vi "TR_Set_List_Item_Value.vi"(8 "error in (no error)":errorcluster, 9 "Basic settings":variant, 10 "Track # in":i32, 11 "MulticolumnListbox in":refnum<vi>) -> (0 "error out":errorcluster, 3 "MulticolumnListbox out":refnum<vi>)   [LabVIEW 2018, in "Tracks Repair.lvlib"]
uses:
  Tracks Repair.lvlib
  SubVi's/Controls/CTL_Basic_cage_settings.ctl
  Tracker.lvlib
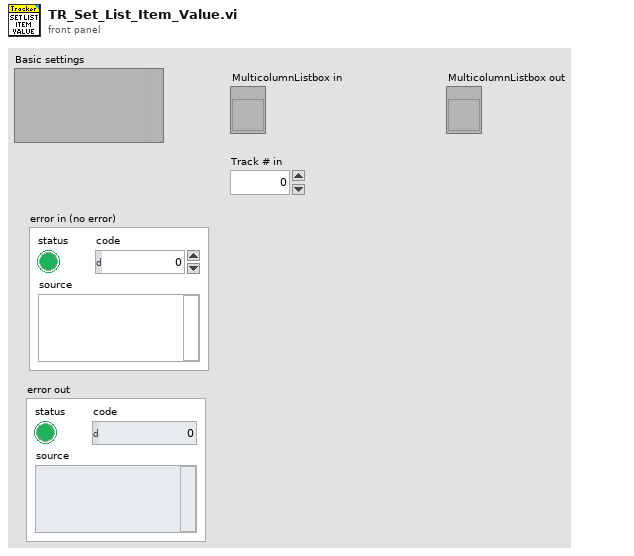
[diagram p1: front panel]
types:
  T1 = typedef "Tracker.lvlib/CTL_Basic_cage_settings.ctl" = cluster{"Vert. offset":dbl, "Hor. offset":dbl, "Bridge swap":bool, "Twisted neck":bool, "Cage diam.":i32, "Magn.rot.":i32, "Acq. speed":dbl}
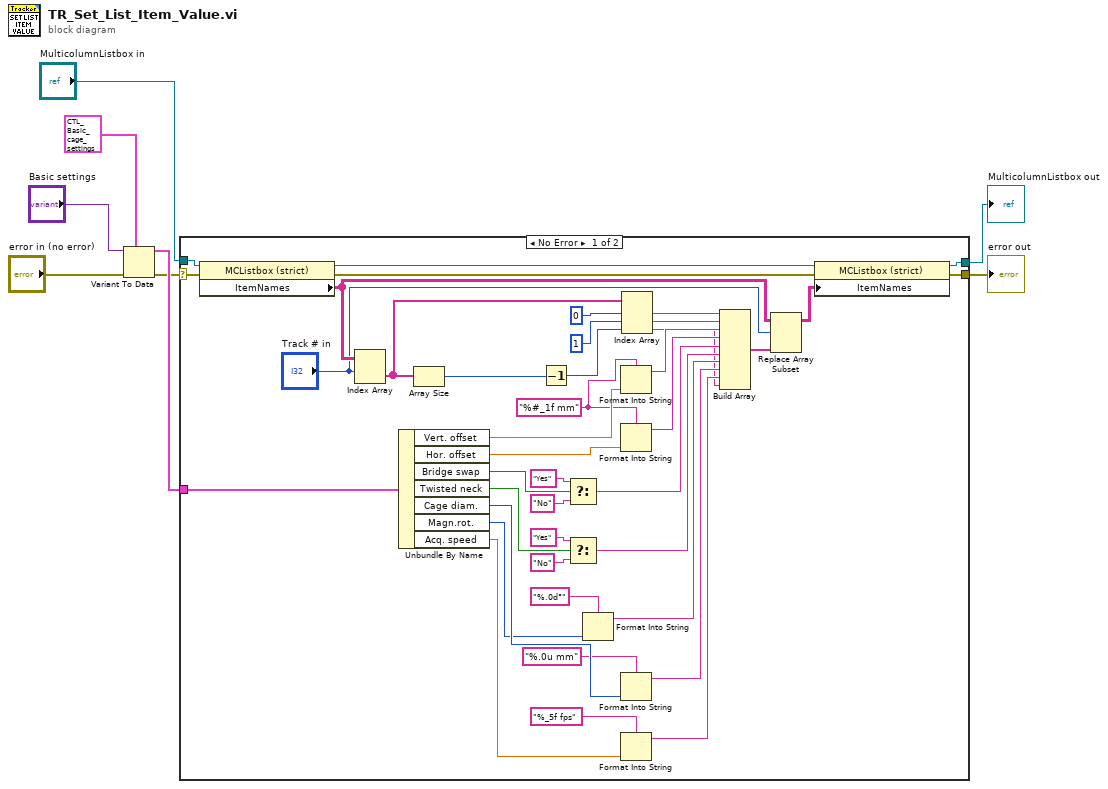
[diagram p0: block diagram]
diagram:
  n1 = Variant To Data(error in="error in (no error)", type=T1 {"Vert. offset"=10.0, "Hor. offset"=0.0, "Bridge swap"=FALSE, "Twisted neck"=FALSE, "Cage diam."=325, "Magn.rot."=0, "Acq. speed"=100.01280589338842} ("Basic settings"), Variant="Basic settings") -> (data=w6:T1, error out=w1:errorcluster)
  n2 = case shown="No Error" w1 {
    selector: w1 -> [w9 w51]
    tunnel: w6 -> [w27 _]
    tunnel: "MulticolumnListbox in" -> [w26 w50]
    tunnel: [w11 w51] -> w3
    tunnel: [w10 w50] -> w2
    frame No Error {
      w30 = "%#_1f mm" ("format string")
      n3 = property class="MCListbox (strict)"(reference=w26, error in=w9) -> (reference out=w13:refnum<vi>, error out=w14:errorcluster, "ItemNames"=w17:string[][])
      n4 = Index Array(array=w17, index (row)="Track # in") -> (element=w22:string[])  [unwired: 1 in]
      n5 = Unbundle By Name(w27) -> ("Vert. offset"=w49:dbl, "Hor. offset"=w47:dbl, "Bridge swap"=w45:bool, "Twisted neck"=w40:bool, "Cage diam."=w37:i32, "Magn.rot."=w35:i32, "Acq. speed"=w33:dbl)
      n6 = Array Size(array=w22) -> (size(s)=w25:i32)
      n7 = Decrement(x=w25) -> (x-1=w24:i32)
      n8 = Select(t="Yes", s=w45, f="No") -> (s? t:f=w39:string)
      n9 = Select(t="Yes", s=w40, f="No") -> (s? t:f=w38:string)
      n10 = Format Into String(format string="%.0d°", w35) -> (resulting string=w29:string)  [unwired: 2 in, 1 out]
      n11 = Format Into String(format string=w30, w49) -> (resulting string=w48:string)  [unwired: 2 in, 1 out]
      n12 = Format Into String(format string=w30, w47) -> (resulting string=w46:string)  [unwired: 2 in, 1 out]
      n13 = Format Into String(format string="%.0u mm", w37) -> (resulting string=w28:string)  [unwired: 2 in, 1 out]
      n14 = Format Into String(format string="%_5f fps", w33) -> (resulting string=w31:string)  [unwired: 2 in, 1 out]
      n15 = Index Array(array=w22, index #1=0 ("index (row)"), index #2=1 ("index"), index #3=w24) -> (element #1=w20:string, element #2=w19:string, element #3=w18:string)
      n16 = Build Array(w20, w19, w48, w46, w39, w38, w29, w28, w31, w18) -> (w15:string[])
      n17 = Replace Array Subset(array=w17, new element=w15, index (row)="Track # in") -> (w12:string[][])  [unwired: 1 in]
      n18 = property class="MCListbox (strict)"(reference=w13, error in=w14, "ItemNames"=w12) -> (reference out=w10:refnum<vi>, error out=w11:errorcluster)
    }
    frame Error {
    }
  }
  "error out" <- w3
  "MulticolumnListbox out" <- w2
